vi "Instrument Mode Setup (LTE).vi"(5 "CLOSE VISA":bool, 6 "SET/GET":string(combo)="GET", 8 "error in":errorcluster {"code" format="%.0x"}, 9 "Select STD BW":string(combo)="RAD:STAN:PRES B10M", 10 "Timeout":u32=3000, 11 "Session In":refnum<visa-resource-name>="GPIB0::18::INSTR") -> (0 "error out":errorcluster {"code" format="%.0x"}, 2 "INST":string, 3 "reference out":refnum<visa-resource-name>)   [LabVIEW 2018]
doc: "Launches the Instrument I/O Assistant, which you can use to communicate with message-based instruments and graphically parse the response. For example you can communicate with an instrument that uses a serial, Ethernet, or GPIB interface."
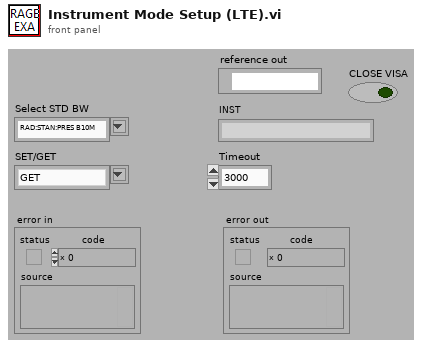
[diagram p1: front panel]
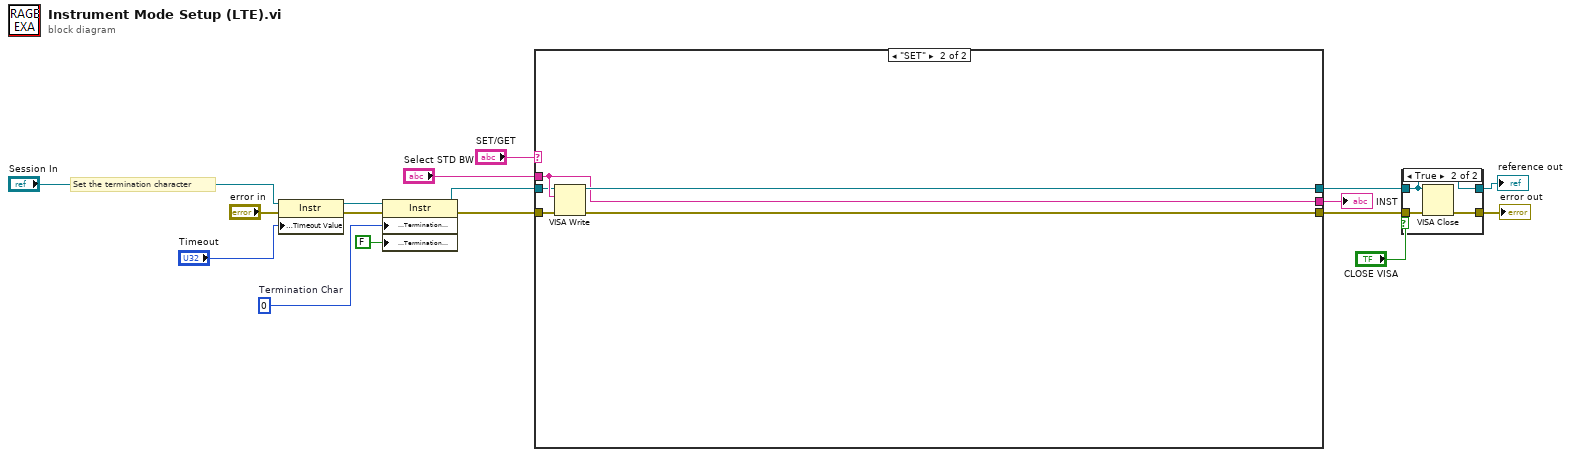
[diagram p0: block diagram]
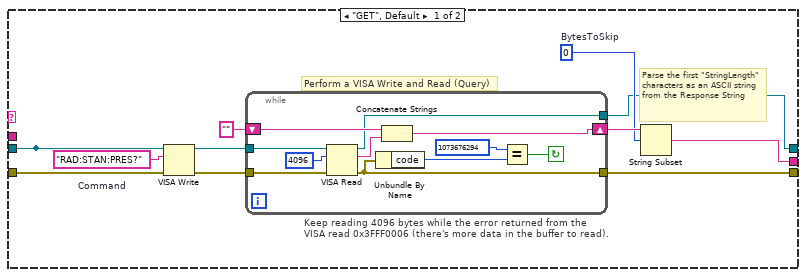
[diagram p3: hidden frame]
diagram:
  w12 = u8 0  # Termination Char
  # "Set the termination character"
  n1 = property class="Instr"(reference="Session In", error in="error in", "General Settings:Timeout Value"="Timeout") -> (reference out=w11:refnum<visa-resource-name>, error out=w14:errorcluster)
  n2 = property class="Instr"(reference=w11, error in=w14, "Message Based Settings:Termination Character"=w12, "Message Based Settings:Termination Character Enable"=FALSE ("enable")) -> (reference out=w1:refnum<visa-resource-name>, error out=w13:errorcluster)
  n3 = case shown="\"SET\"" "SET/GET" {
    tunnel: w13 -> [w28 w44]
    tunnel: [w25 w43] -> w7
    tunnel: [w23 w41] -> w9
    tunnel: [w18 w40] -> _
    tunnel: "Select STD BW" -> [_ w41]
    tunnel: [w20 w42] -> w3
    tunnel: w1 -> [w18 w40]
    frame "GET", Default {
      w21 = 0  # BytesToSkip
      w19 = "RAD:STAN:PRES?"  # Command
      # "Parse the first \"StringLength\" characters as an ASCII string from the Response String"
      # "Perform a VISA Write and Read (Query)"
      # "Keep reading 4096 bytes while the error returned from the\nVISA read 0x3FFF0006 (there's more data in the buffer to read)."
      n4 = VISA Write(VISA resource name=w18, write buffer=w19, error in (no error)=w28) -> (VISA resource name out=w27:refnum<visa-resource-name>, error out=w26:errorcluster)  [unwired: 1 out]
      n5 = while {
        tunnel: w27 -> [w36]
        shift-right: [w30] -> w22
        shift-left: "" -> [w35]
        tunnel: w26 -> [w33]
        tunnel: [w32] -> w25
        tunnel: [w29] -> w20
        stop <- w31 continue-if-true
        n6 = VISA Read(VISA resource name=w36, byte count=u32 4096 ("byte count (0)"), error in (no error)=w33) -> (VISA resource name out=w29:refnum<visa-resource-name>, read buffer=w34:string, error out=w32:errorcluster)  [unwired: 1 out]
        n7 = Unbundle By Name(w32) -> ("code"=w38:i32)
        n8 = Concatenate Strings(w35, w34) -> (w30:string)
        n9 = Equal?(x=1073676294, y=w38) -> (x = y?=w31:bool)
      }
      n10 = String Subset(string=w22, offset (0)=w21) -> (substring=w23:string)  [unwired: 1 out]
    }
    frame "SET" {
      n11 = VISA Write(VISA resource name=w40, write buffer=w41, error in (no error)=w44) -> (VISA resource name out=w42:refnum<visa-resource-name>, error out=w43:errorcluster)  [unwired: 1 out]
    }
  }
  "INST" <- w9
  n12 = case shown="True" "CLOSE VISA" {
    tunnel: w3 -> [w45 w47]
    tunnel: w7 -> [w46 w49]
    tunnel: [w46 w48] -> w6
    tunnel: [w45 w47] -> w2
    frame False {
    }
    frame True {
      n13 = VISA Close(VISA resource name=w47, error in (no error)=w49) -> (error out=w48:errorcluster)
    }
  }
  "error out" <- w6
  "reference out" <- w2
